vi "Set software shutter.vi"(8 "error in (no error)":errorcluster, 9 "Imaging Protocol":T1, 11 "Acquired z-plane index":i32) -> (0 "Error Out":errorcluster)   [LabVIEW 2017]
uses:
  Typedefs/Imaging Protocols enum.ctl
  Global Variables/General Globals.vi
  Global Variables/gl_UI Ctrl Refs.vi
  Pockels/Globals/gl_Pockels control globals.vi
panel:
  out "Execution time (ms)":u32
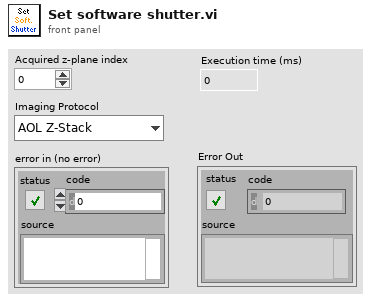
[diagram p1: front panel]
types:
  T1 = typedef "Imaging Protocols enum.ctl" = enum16{"AOL Z-Stack", "Motor Z Stack", "Functional Acquisition", "Single Plane Acquisition", "Volume Acquisition", "Live Imaging", "Live Plane Imaging", "Live Volume Imaging"}
  T2 = typedef "UI ctrl refs cluster.ctl" = cluster{"Top level VI path":path, "Top level VI ref":refnum<vi>, "User menu ref":refnum<k9>, "Sub Panel control":refnum<vi>, "Imaging Param Tab":refnum<vi>, "Occurrence-Start drivers":refnum<k4>, "Occurrence-Speed logging initialised":refnum<k4>, "Occurrence-XYZ stage initialised":refnum<k4>, "Exit button":refnum<vi>, "Status ind":refnum<vi>, "Set as origin":refnum<vi>, "Speed Logging":refnum<vi>, "Time Lapse":refnum<vi>, "Live Imaging":refnum<vi>, "AOL Z Stack":refnum<vi>, "Motor Z Stack":refnum<vi>, "Funct Acq button":refnum<vi>, "Hard Shutter":refnum<vi>, "Virtual Shutter":refnum<vi>, "Laser Power":refnum<vi>, "AOL Mode":refnum<vi>, "Frame Size":refnum<vi>, "Field of View":refnum<vi>, "Dwell Time":refnum<vi>, "Zoom":refnum<vi>, "AOL Z":refnum<vi>, "Objective":refnum<vi>, "Axis":refnum<vi>, "Paths & Names":refnum<vi>, "Experiment folder path (ind.)":refnum<vi>, "Last State (Ind.)":refnum<vi>, "Laser wavelength ind (nm)":refnum<vi>, "Averages":refnum<vi>, "Angle (degrees)":refnum<vi>, "X centre":refnum<vi>, "Y centre":refnum<vi>, "Plane Mode":refnum<vi>, "# Planes":refnum<vi>, "Z Start":refnum<vi>, "Z Stop":refnum<vi>, "Z Step":refnum<vi>, "PMT 1":refnum<vi>, "PMT 2":refnum<vi>, "Stage XYZ Position":refnum<vi>, "Pockels@Z Start":refnum<vi>, "Pockels@Z Stop":refnum<vi>, "Obtain Z Start":refnum<vi>, "Obtain Z Stop":refnum<vi>, "Live stim.trig.period":refnum<vi>, "Live stim.trig.enable":refnum<vi>, "Movement Correction":refnum<vi>, "Load Reference Image":refnum<vi>, "XY Stage Move":refnum<vi>, "MovCor Cluster":refnum<vi>, "RefDAQParam":refnum<vi>, "Funct. Acq. Pockels Modulation":refnum<vi>, "Background MovCor":refnum<vi>, "Ref Laser Power":refnum<vi>, "Enable Video Recording":refnum<vi>, "Video Record-Live Imaging":refnum<vi>, "Video Record-Funct acq":refnum<vi>, "Reference Source":refnum<vi>, "AOL Z-stack Chirps Ready (ind)":refnum<vi>, "Target time between mov.cor. ref triggers (ms)":refnum<vi>, "Funct. Acq. Ref frame save":refnum<vi>, "Tracking button":refnum<vi>, "Show ref plots window":refnum<vi>, "Center freq ind (nm)":refnum<vi>, "Pickup mode (ind)":refnum<vi>, "Logging queue (ind)":refnum<vi>, "Back aperture power (ind.)":refnum<vi>, "Power after objective (ind.)":refnum<vi>, "Switch user":refnum<vi>}
  T3 = typedef "Laser control knob.ctl" = u16
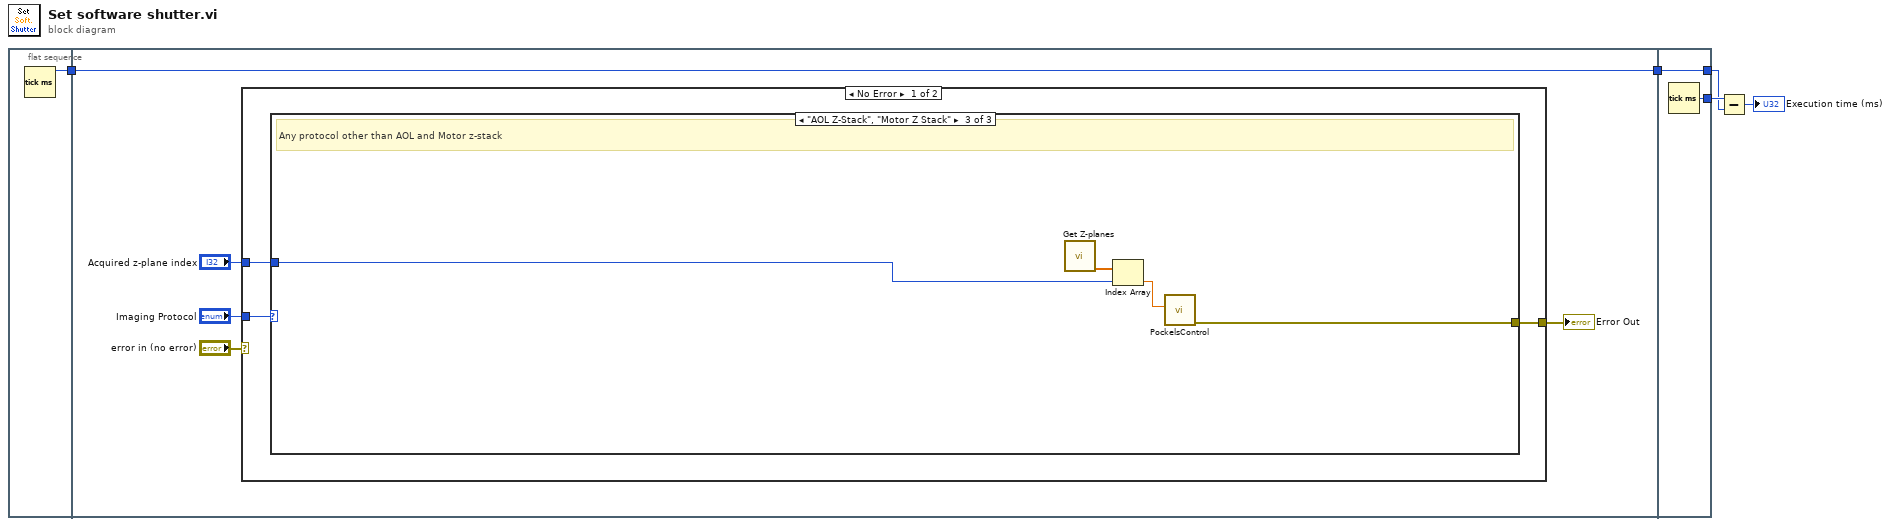
[diagram p0: block diagram]
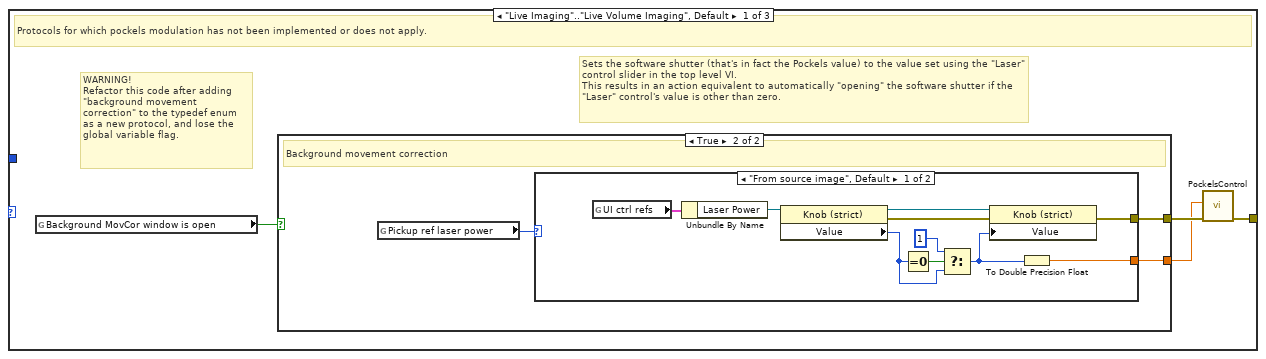
[diagram p2: hidden frame]
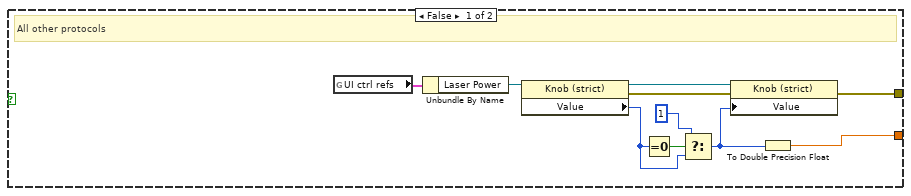
[diagram p3: hidden frame]
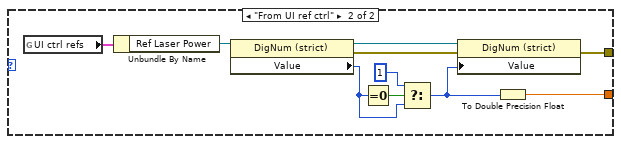
[diagram p4: hidden frame]
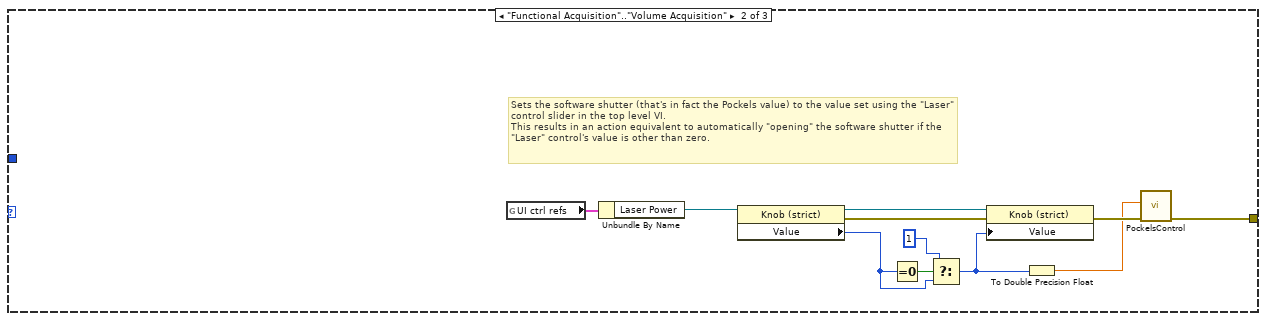
[diagram p5: hidden frame]
diagram:
  n1 = flat-sequence {
    tunnel: [w6] -> w4
    tunnel: w4 -> [w7]
    tunnel: [w7] -> w3
    tunnel: [w69] -> w5
    tunnel: w3 -> [w68]
    tunnel: [w68] -> w2
    frame #0 {
      n2 = Tick Count (ms)() -> (millisecond timer value=w6:u32)
    }
    frame #1 {
      n3 = case shown="No Error" "error in (no error)" {
        selector: "error in (no error)" -> [_ w67]
        tunnel: "Imaging Protocol" -> [w13 _]
        tunnel: "Acquired z-plane index" -> [w14 _]
        tunnel: [w12 w67] -> w8
        frame No Error {
          n4 = case shown="\"AOL Z-Stack\", \"Motor Z Stack\"" w13 {
            tunnel: [w17 w52 w63] -> w12
            tunnel: w14 -> [_ _ w65]
            frame "Live Imaging".."Live Volume Imaging", Default {
              # "WARNING!\nRefactor this code after adding \"background movement correction\" to the typedef enum as a new protocol, and lose the global variable flag."
              # "Sets the software shutter (that's in fact the Pockels value) to the value set using the \"Laser\" control slider in the top level VI. \nThis results in an action equivalent to automatically \"opening\" the software shutter if the \"Laser\" control's value is other than zero."
              # "Protocols for which pockels modulation has not been implemented or does not apply."
              n5 = global read "General Globals.vi" "Background MovCor window is open"() -> (w15:bool)
              n6 = case shown="True" w15 {
                tunnel: [w22 w31] -> w18
                tunnel: [w21 w30] -> w16
                frame False {
                  # "All other protocols"
                  n7 = global read "gl_UI Ctrl Refs.vi" "UI ctrl refs"() -> (w20:T2)
                  n8 = Unbundle By Name(w20) -> ("Laser Power"=w19:refnum<vi>)
                  n9 = property class="Knob (strict)"(reference=w19) -> (reference out=w25:refnum<vi>, error out=w24:errorcluster, "Value"=w26:T3)  [unwired: 1 in]
                  n10 = Equal To 0?(x=w26) -> (x = 0?=w28:bool)
                  n11 = Select(t=u16 1, s=w28, f=w26) -> (s? t:f=w23:T3)
                  n12 = property class="Knob (strict)"(reference=w25, error in=w24, "Value"=w23) -> (error out=w22:errorcluster)  [unwired: 1 out]
                  n13 = To Double Precision Float(number=w23) -> (double precision float=w21:dbl)
                }
                frame True {
                  # "Background movement correction"
                  n14 = global read "gl_Pockels control globals.vi" "Pickup ref laser power"() -> (w29:enum16{"From source image", "From UI ref ctrl"})
                  n15 = case shown="\"From source image\", Default" w29 {
                    tunnel: [w32 w45] -> w31
                    tunnel: [w33 w44] -> w30
                    frame "From source image", Default {
                      n16 = global read "gl_UI Ctrl Refs.vi" "UI ctrl refs"() -> (w35:T2)
                      n17 = Unbundle By Name(w35) -> ("Laser Power"=w34:refnum<vi>)
                      n18 = property class="Knob (strict)"(reference=w34) -> (reference out=w38:refnum<vi>, error out=w37:errorcluster, "Value"=w39:T3)  [unwired: 1 in]
                      n19 = Equal To 0?(x=w39) -> (x = 0?=w41:bool)
                      n20 = Select(t=u16 1, s=w41, f=w39) -> (s? t:f=w36:T3)
                      n21 = property class="Knob (strict)"(reference=w38, error in=w37, "Value"=w36) -> (error out=w32:errorcluster)  [unwired: 1 out]
                      n22 = To Double Precision Float(number=w36) -> (double precision float=w33:dbl)
                    }
                    frame "From UI ref ctrl" {
                      n23 = global read "gl_UI Ctrl Refs.vi" "UI ctrl refs"() -> (w42:T2)
                      n24 = Unbundle By Name(w42) -> ("Ref Laser Power"=w43:refnum<vi>)
                      n25 = property class="DigNum (strict)"(reference=w43) -> (reference out=w48:refnum<vi>, error out=w47:errorcluster, "Value"=w49:u8)  [unwired: 1 in]
                      n26 = Equal To 0?(x=w49) -> (x = 0?=w51:bool)
                      n27 = Select(t=u16 1, s=w51, f=w49) -> (s? t:f=w46:u16)
                      n28 = property class="DigNum (strict)"(reference=w48, error in=w47, "Value"=w46) -> (error out=w45:errorcluster)  [unwired: 1 out]
                      n29 = To Double Precision Float(number=w46) -> (double precision float=w44:dbl)
                    }
                  }
                }
              }
              n30 = call "PockelsControl.vi"("Error In"=w18, "Laser Power (%)"=w16) -> ("Error Out"=w17:errorcluster)  [unwired: 9 in]
            }
            frame "Functional Acquisition".."Volume Acquisition" {
              # "Sets the software shutter (that's in fact the Pockels value) to the value set using the \"Laser\" control slider in the top level VI. \nThis results in an action equivalent to automatically \"opening\" the software shutter if the \"Laser\" control's value is other than zero."
              n31 = global read "gl_UI Ctrl Refs.vi" "UI ctrl refs"() -> (w62:T2)
              n32 = Unbundle By Name(w62) -> ("Laser Power"=w61:refnum<vi>)
              n33 = property class="Knob (strict)"(reference=w61) -> (reference out=w57:refnum<vi>, error out=w56:errorcluster, "Value"=w58:T3)  [unwired: 1 in]
              n34 = Equal To 0?(x=w58) -> (x = 0?=w60:bool)
              n35 = Select(t=u16 1, s=w60, f=w58) -> (s? t:f=w55:T3)
              n36 = property class="Knob (strict)"(reference=w57, error in=w56, "Value"=w55) -> (error out=w54:errorcluster)  [unwired: 1 out]
              n37 = To Double Precision Float(number=w55) -> (double precision float=w53:dbl)
              n38 = call "PockelsControl.vi"("Error In"=w54, "Laser Power (%)"=w53) -> ("Error Out"=w52:errorcluster)  [unwired: 9 in]
            }
            frame "AOL Z-Stack", "Motor Z Stack" {
              # "Any protocol other than AOL and Motor z-stack"
              n39 = call "Get Z-planes.vi"() -> ("Pockels vs. Z (Laser power %)"=w66:dbl[])  [unwired: 7 in, 4 out]
              n40 = Index Array(array=w66, index=w65) -> (element=w64:dbl)
              n41 = call "PockelsControl.vi"("Laser Power (%)"=w64) -> ("Error Out"=w63:errorcluster)  [unwired: 10 in]
            }
          }
        }
        frame Error {
        }
      }
      "Error Out" <- w8
    }
    frame #2 {
      n42 = Tick Count (ms)() -> (millisecond timer value=w69:u32)
    }
  }
  n43 = Subtract(x=w5, y=w2) -> (x-y=→"Execution time (ms)":u32)
